vi "Create Log File.vi"(8 "error in (no error)":errorcluster, 10 "LogHeader String":string, 11 "LogFile Folder":path) -> (0 "error out":errorcluster, 3 "new file path":path)   [LabVIEW 2020]
doc: "Developed by Kevin Thompson\nkevin@thompsonengineering.net\n\nCopyright 2018-2020\nThompson Engineering, LLC"
uses:
  <userlib>/_OpenG.lib/file/file.llb/File Exists - Scalar__ogtk.vi
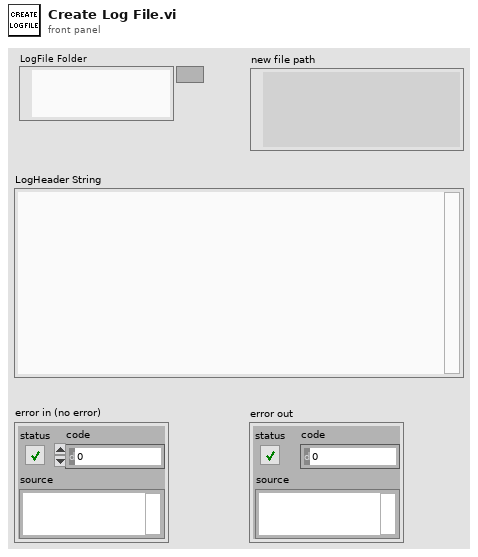
[diagram p1: front panel]
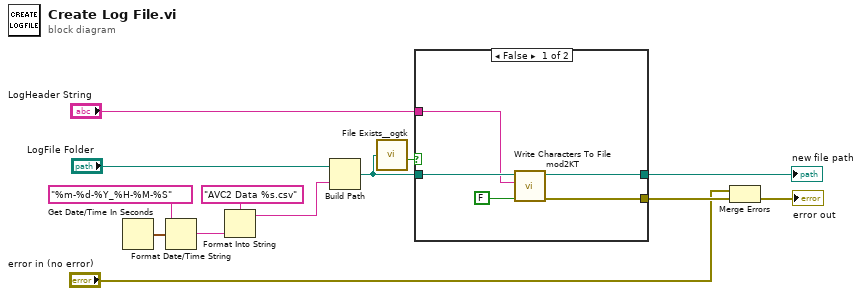
[diagram p0: block diagram]
diagram:
  n1 = Get Date/Time In Seconds() -> (seconds since 1Jan1904=w8:timestamp)
  n2 = Format Date/Time String(time format string (%c)="%m-%d-%Y_%H-%M-%S", seconds (now)=w8) -> (date/time string=w9:string)  [unwired: 1 in]
  n3 = Format Into String(format string="AVC2 Data %s.csv", w9) -> (resulting string=w11:string)  [unwired: 2 in, 1 out]
  n4 = Build Path(base path="LogFile Folder", name or relative path=w11) -> (appended path=w13:path)
  n5 = call-poly <userlib>:"File Exists__ogtk.vi"("file path"=w13) -> ("exists"=w12:bool)  [unwired: 6 in, 1 out]
  n6 = case shown="False" w12 {
    tunnel: w13 -> [w18 w19]
    tunnel: [w16 w19] -> w6
    tunnel: [w15 _] -> w5
    tunnel: "LogHeader String" -> [w14 _]
    frame False {
      n7 = call <vilib>:"Write Characters To File mod2KT.vi"("append to file? (new file:F)"=FALSE, "character string"=w14, "file path (dialog if empty)"=w18) -> ("error out"=w15:errorcluster, "new file path (Not A Path if cancelled)"=w16:path)  [unwired: 3 in]
    }
    frame True {
    }
  }
  "new file path" <- w6
  n8 = Merge Errors("error in (no error)", w5) -> (→"error out":errorcluster)
